vi "decodeObject.vi"(8 "error in (no error)":errorcluster, 10 "ByteArray":u8[](array[numeric])) -> (0 "error out":errorcluster, 1 "Variant":variant, 2 "RemainingBytes":u8[](array[numeric]), 3 "Type":string)   [LabVIEW 2016, in "MsgPack.lvlib"]
uses:
  MsgPack.lvlib
  <vilib>/Utility/error.llb/Error Cluster From Error Code.vi
  <vilib>/ErrorRing/Error Ring.xnode
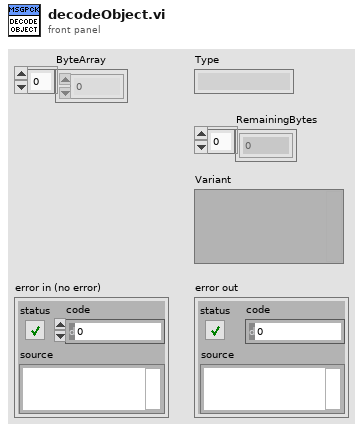
[diagram p1: front panel]
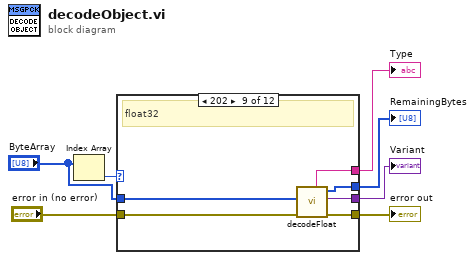
[diagram p0: block diagram]
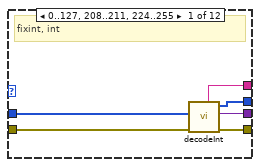
[diagram p2: hidden frame]
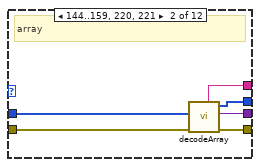
[diagram p3: hidden frame]
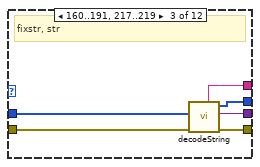
[diagram p4: hidden frame]
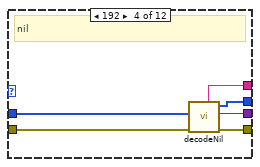
[diagram p5: hidden frame]
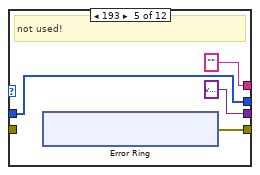
[diagram p6: hidden frame]
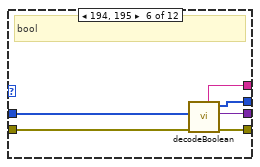
[diagram p7: hidden frame]
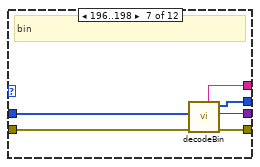
[diagram p8: hidden frame]
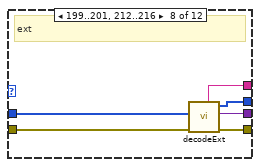
[diagram p9: hidden frame]
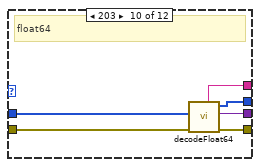
[diagram p10: hidden frame]
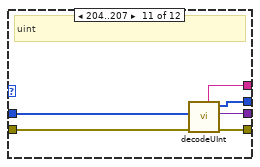
[diagram p11: hidden frame]
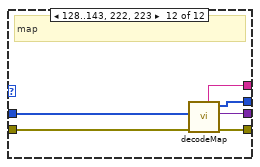
[diagram p12: hidden frame]
diagram:
  n1 = Index Array(array="ByteArray") -> (element=w7:u8)  [unwired: 1 in]
  n2 = case shown="202" w7 {
    tunnel: "ByteArray" -> [w13 w18 w25 w28 w32 w46 w52 w58 w64 w70 w76 w82]
    tunnel: [w11 w16 w23 w31 w35 w44 w50 w56 w62 w68 w74 w78] -> w1
    tunnel: [w12 w15 w24 w30 variant ("variant") w45 w51 w57 w63 w69 w75 w80] -> w5
    tunnel: "error in (no error)" -> [w10 w19 w20 w29 _ w43 w47 w53 w59 w65 w71 w81]
    tunnel: [w9 w17 w22 w27 w32 w41 w49 w55 w61 w66 w72 w79] -> w2
    tunnel: [w8 w14 w21 w26 "" ("Type") w42 w48 w54 w60 w67 w73 w77] -> w3
    frame 0..127, 208..211, 224..255 {
      # "fixint, int"
      n3 = call "decodeInt.vi"("error in (no error)"=w10, "ByteArray"=w13) -> ("error out"=w11:errorcluster, "variant"=w12:variant, "RemainingBytes"=w9:u8[], "Type"=w8:string)  [unwired: 5 in, 1 out]
    }
    frame 144..159, 220, 221 {
      # "array"
      n4 = call "decodeArray.vi"("error in (no error)"=w19, "ByteArray"=w18) -> ("error out"=w16:errorcluster, "variant"=w15:variant, "ByteArray"=w17:u8[], "Type"=w14:string)  [unwired: 6 in]
    }
    frame 160..191, 217..219 {
      # "fixstr, str"
      n5 = call "decodeString.vi"("error in (no error)"=w20, "ByteArray"=w25) -> ("error out"=w23:errorcluster, "variant"=w24:variant, "RemainingBytes"=w22:u8[], "Type"=w21:string)  [unwired: 5 in, 1 out]
    }
    frame 192 {
      # "nil"
      n6 = call "decodeNil.vi"("error in (no error)"=w29, "ByteArray"=w28) -> ("error out"=w31:errorcluster, "variant"=w30:variant, "RemainingBytes"=w27:u8[], "Type"=w26:string)  [unwired: 6 in]
    }
    frame 193 {
      # "not used!"
      n7 = xnode "Error Ring"() -> ("Fehler (Ausgang)"=w35:errorcluster)
    }
    frame 194, 195 {
      # "bool"
      n8 = call "decodeBoolean.vi"("error in (no error)"=w43, "ByteArray"=w46) -> ("error out"=w44:errorcluster, "variant"=w45:variant, "RemainingBytes"=w41:u8[], "Type"=w42:string)  [unwired: 5 in, 1 out]
    }
    frame 196..198 {
      # "bin"
      n9 = call "decodeBin.vi"("error in (no error)"=w47, "ByteArray"=w52) -> ("error out"=w50:errorcluster, "variant"=w51:variant, "RemainingBytes"=w49:u8[], "Type"=w48:string)  [unwired: 5 in, 1 out]
    }
    frame 199..201, 212..216 {
      # "ext"
      n10 = call "decodeExt.vi"("error in (no error)"=w53, "ByteArray"=w58) -> ("error out"=w56:errorcluster, "variant"=w57:variant, "RemainingBytes"=w55:u8[], "Type"=w54:string)  [unwired: 5 in, 1 out]
    }
    frame 202 {
      # "float32"
      n11 = call "decodeFloat.vi"("error in (no error)"=w59, "ByteArray"=w64) -> ("error out"=w62:errorcluster, "variant"=w63:variant, "RemainingBytes"=w61:u8[], "Type"=w60:string)  [unwired: 5 in, 1 out]
    }
    frame 203 {
      # "float64"
      n12 = call "decodeFloat64.vi"("error in (no error)"=w65, "ByteArray"=w70) -> ("error out"=w68:errorcluster, "variant"=w69:variant, "RemainingBytes"=w66:u8[], "Type"=w67:string)  [unwired: 5 in, 1 out]
    }
    frame 204..207 {
      # "uint"
      n13 = call "decodeUInt.vi"("error in (no error)"=w71, "ByteArray"=w76) -> ("error out"=w74:errorcluster, "variant"=w75:variant, "RemainingBytes"=w72:u8[], "Type"=w73:string)  [unwired: 5 in, 1 out]
    }
    frame 128..143, 222, 223 {
      # "map"
      n14 = call "decodeMap.vi"("error in (no error)"=w81, "ByteArray"=w82) -> ("error out"=w78:errorcluster, "variant"=w80:variant, "ByteArray"=w79:u8[], "Type"=w77:string)  [unwired: 6 in]
    }
  }
  "Variant" <- w5
  "Type" <- w3
  "RemainingBytes" <- w2
  "error out" <- w1
